vi "Create Query (from Variant Attributes).vi"(5 "URI-Component.Query":refnum<class "URI-Component.Query.lvclass">, 8 "error in (no error)":errorcluster, 11 "Query":variant) -> (0 "error out":errorcluster, 3 "URI-Component.Query":refnum<class "URI-Component.Query.lvclass">)   [LabVIEW 2013, in "openURI.lvlib" / "URI-Component.Query.lvclass"]
uses:
  URI-Component.Query.lvclass
  URI-Component.Query.lvclass/URI-Component.Query.ctl
  <vilib>/ErrorRing/Error Ring.xnode
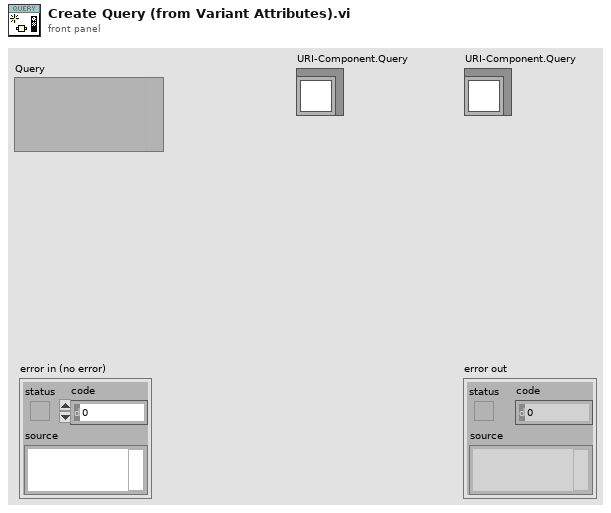
[diagram p1: front panel]
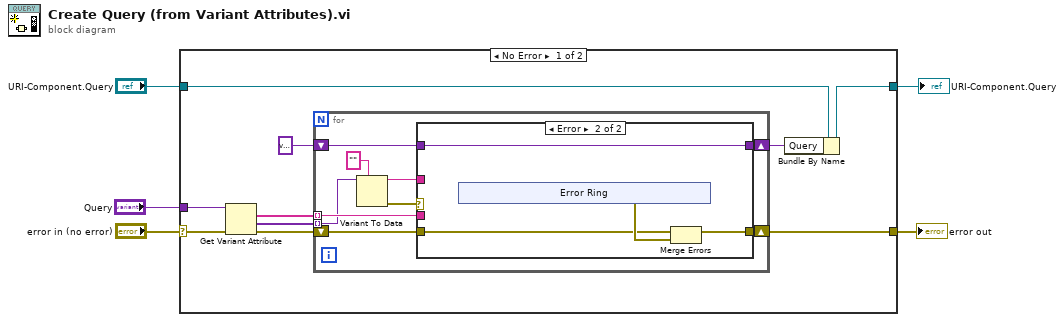
[diagram p0: block diagram]
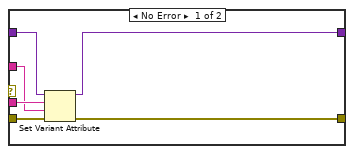
[diagram p2: hidden frame]
diagram:
  n1 = case shown="No Error" "error in (no error)" {
    selector: "error in (no error)" -> [w7 w37]
    tunnel: [w6 w37] -> w4
    tunnel: [w14 w36] -> w2
    tunnel: "URI-Component.Query" -> [w15 w36]
    tunnel: "Query" -> [w9 _]
    frame No Error {
      n2 = Get Variant Attribute(Variant=w9, error in=w7) -> (names=w12:string[], values=w11:variant[], error out=w13:errorcluster)  [unwired: 2 in, 1 out]
      n3 = for {
        shift-right: [w22] -> w6
        shift-left: w13 -> [w23]
        shift-right: [w24] -> w8
        shift-left: variant ("Query") -> [w21]
        tunnel: w12 -> [w20] mode=indexing
        tunnel: w11 -> [w19] mode=indexing
        n4 = Variant To Data(type="", Variant=w19) -> (data=w16:string, error out=w18:errorcluster)  [unwired: 1 in]
        n5 = case shown="Error" w18 {
          tunnel: [w30 w34] -> w24
          tunnel: w23 -> [w29 w32]
          tunnel: [w28 w31] -> w22
          tunnel: w21 -> [w27 w34]
          tunnel: w20 -> [w26 _]
          tunnel: w16 -> [w25 _]
          frame No Error {
            n6 = Set Variant Attribute(Variant=w27, name=w26, value=w25, error in=w29) -> (Variant out=w30:variant, error out=w28:errorcluster)  [unwired: 1 out]
          }
          frame Error {
            n7 = xnode "Error Ring"() -> ("error out"=w33:errorcluster)
            n8 = Merge Errors(w32, w33) -> (w31:errorcluster)
          }
        }
      }
      n9 = Bundle By Name(cluster=w15, "Query"=w8) -> (w14:refnum<class "URI-Component.Query.lvclass">)
    }
    frame Error {
    }
  }
  "error out" <- w4
  "URI-Component.Query" <- w2
